vi "init peaks.vi"(8 "error in":errorcluster, 10 "element":cluster{"Locations":dbl[], "Amplitudes":dbl[]}, 11 "Spectrum":refnum<vi>) -> (0 "error out":errorcluster, 1 "List Parameter Fit Out":dbl[][](array[numeric]), 2 "List ROI Out":dbl[][](array[numeric]), 3 "Peaks Out":cluster{"Locations":dbl[], "Amplitudes":dbl[]}, 4 "Table":string[][](table))   [LabVIEW 2023]
uses:
  e8004514-cfb5-4b90-ae77-451f506fadd8.vi
  <vilib>/Utility/Data Type/Get Array Information.vi
  <vilib>/Utility/Data Type/Get Type Information.vi
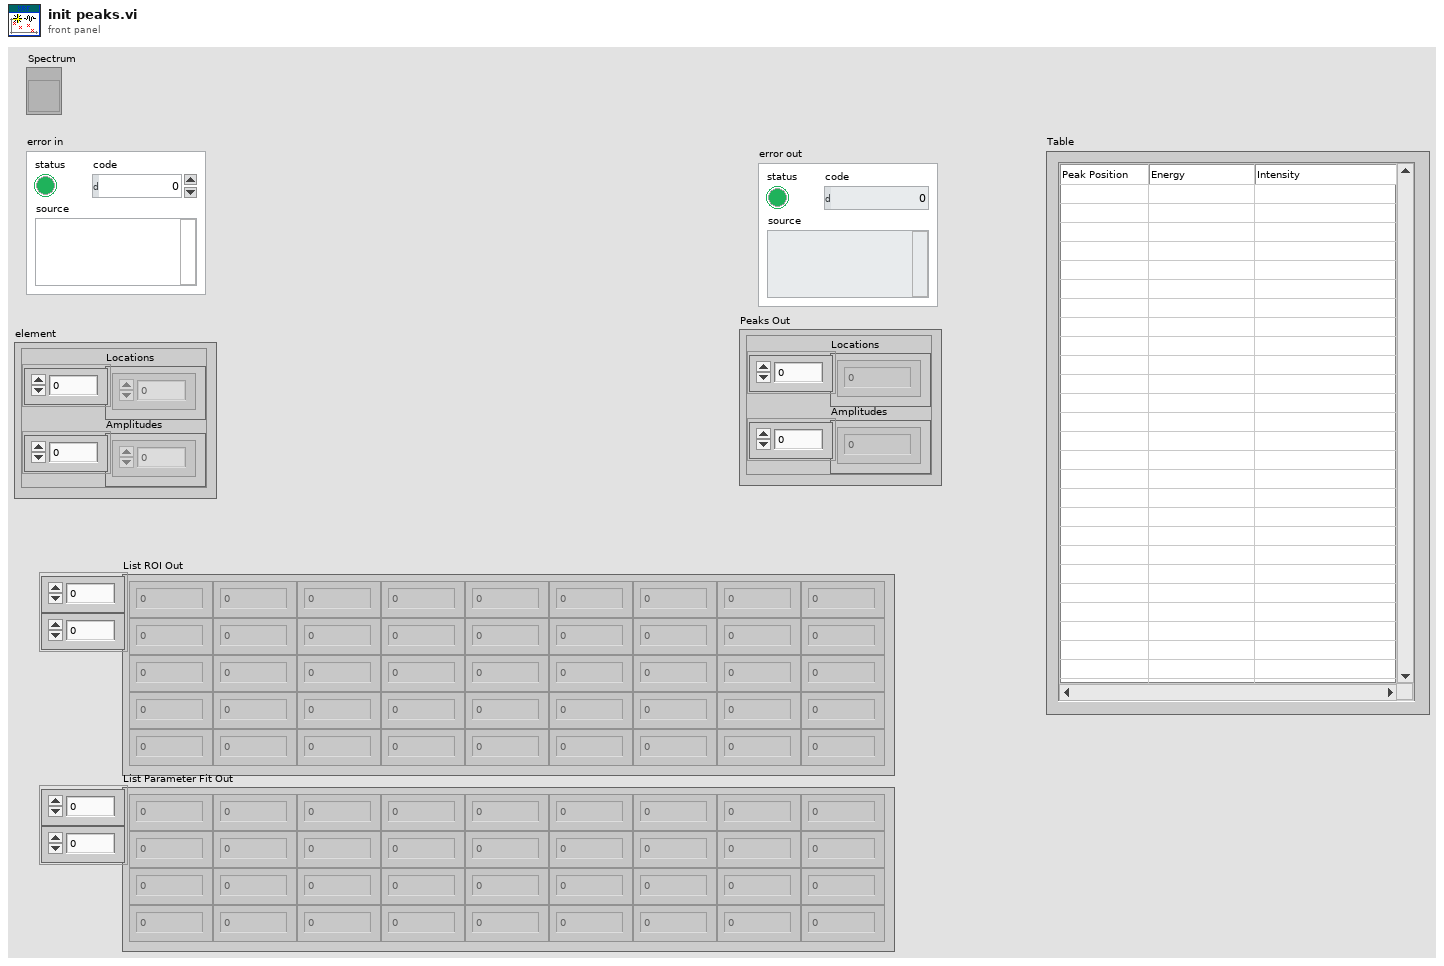
[diagram p1: front panel]
types:
  T1 = typedef "LVCursorListTypeDef.ctl" = cluster{"Name":string, "Color":u32, "Style":u8, "Point Style":u8, "Name Visible":bool, "Allow Drag":bool, "Cursor Mode":u32, "Plot":i32, "Index":i32, "Position":cluster{"X":dbl, "Y":dbl}, "X Scale":u32, "Y Scale":u32, "Watch Plots":i32[], "Watch All Plots":bool, "Plot Area":i32, "Label Offset":cluster{"X":dbl, "Y":dbl}}[]
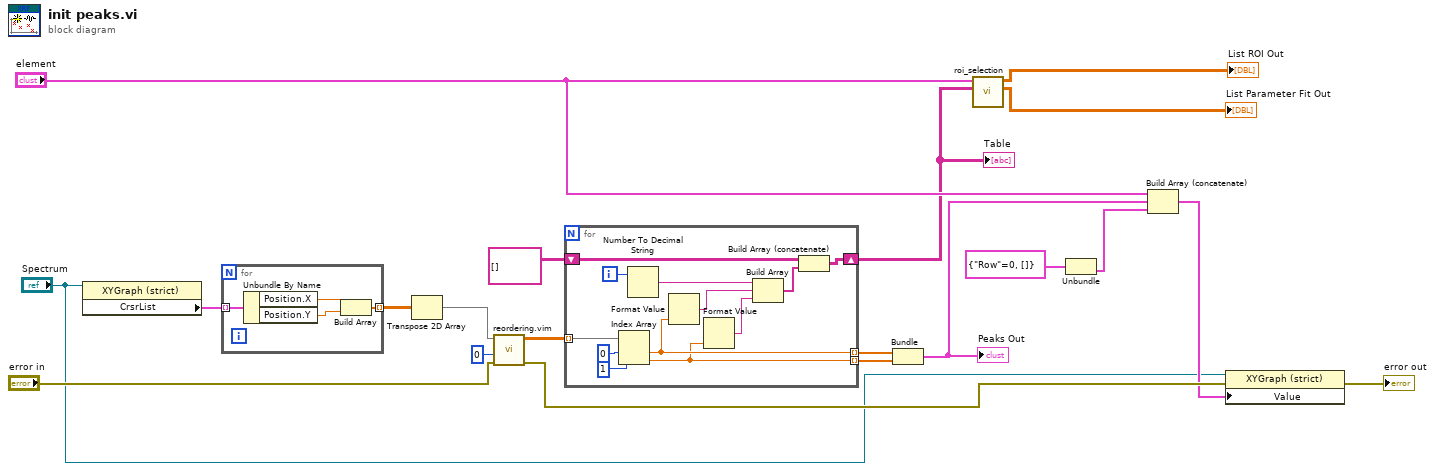
[diagram p0: block diagram]
diagram:
  n1 = property on="Property Node" class="XYGraph (strict)"(reference="Spectrum") -> ("CrsrList"=w12:T1)  [unwired: 1 in, 2 out]
  n2 = for {
    tunnel: w12 -> [w24] mode=indexing
    tunnel: [w21] -> w19 mode=indexing
    n3 = Unbundle By Name(w24) -> ("Position.X"=w23:dbl, "Position.Y"=w22:dbl)
    n4 = Build Array(w23, w22) -> (w21:dbl[])
  }
  n5 = Transpose 2D Array(2D array=w19) -> (transposed array=w18:dbl[][])
  n6 = call "reordering.vim"("error in (no error)"="error in", "Row to Reorder"=0, "Data In"=w18) -> ("Error Out"=w8:errorcluster, "Data Out"=w16:dbl[][])  [unwired: 7 in]
  n7 = for {
    tunnel: w16 -> [w36] mode=indexing
    tunnel: [w32] -> w14 mode=indexing
    tunnel: [w31] -> w13 mode=indexing
    shift-right: [w25] -> w1
    shift-left: string[][] [] ("Table") -> [w27]
    i -> [w33]
    n8 = Index Array(array=w36, index #1=0 ("index"), index #2=1 ("index")) -> (element #1=w32:dbl, element #2=w31:dbl)
    n9 = Number To Decimal String(number=w33) -> (decimal integer string=w28:string)  [unwired: 1 in]
    n10 = Format Value(value (0)=w32) -> (output string=w29:string)  [unwired: 2 in]
    n11 = Format Value(value (0)=w31) -> (output string=w30:string)  [unwired: 2 in]
    n12 = Build Array(w28, w29, w30) -> (w26:string[])
    n13 = Build Array (concatenate)(w27, w26) -> (w25:string[][])
  }
  "Table" <- w1
  n14 = Bundle(w14, w13) -> (w4:cluster{dbl[], dbl[]})  [unwired: 1 in]
  "Peaks Out" <- w4
  n15 = call "roi_selection.vi"("List Peaks"=w1, "Spectrum In"="element") -> ("List Parameter Fit Out"=→"List Parameter Fit Out":dbl[][], "List ROI Out"=→"List ROI Out":dbl[][])  [unwired: 8 in]
  n16 = Unbundle(cluster{"Row":i32, cluster{dbl[], dbl[]}[]} {"Row"=0, []}) -> (w5:cluster{dbl[], dbl[]}[])  [unwired: 1 out]
  n17 = Build Array (concatenate)("element", w4, w5) -> (w3:cluster{"Locations":dbl[], "Amplitudes":dbl[]}[])
  n18 = property on="Property Node" class="XYGraph (strict)"(reference="Spectrum", error in=w8, "Value"=w3) -> (error out=→"error out":errorcluster)  [unwired: 1 out]
